vi "Calibration.vi"() -> ()   [LabVIEW 2014]
uses:
  <vilib>/vision/Vision Builder AI/API.llb/IVB Interface - VBAI Version.ctl
panel:
  out "error out":errorcluster
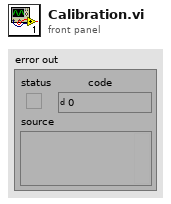
[diagram p1: front panel]
types:
  T1 = typedef "IVB Interface - VBAI Version.ctl" = u16
  T2 = enum32{"invalid app kind", "Development System", "Run Time System", "Student Edition", "Embedded LabVIEW", "Evaluation", "Custom"}
  T3 = typedef "VBAIInterface.ctl" = refnum<k21>
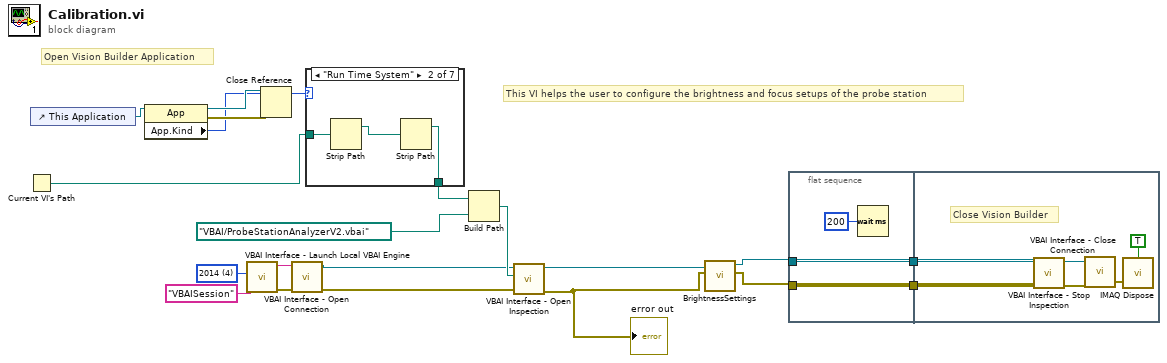
[diagram p0: block diagram]
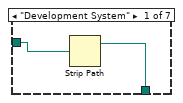
[diagram p2: hidden frame]
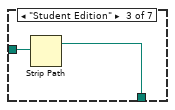
[diagram p3: hidden frame]
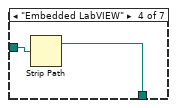
[diagram p4: hidden frame]
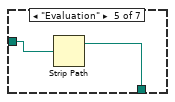
[diagram p5: hidden frame]
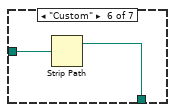
[diagram p6: hidden frame]
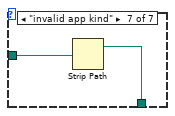
[diagram p7: hidden frame]
diagram:
  w20 = T1 4 items=["2010", "2011", "2012", "2013", "2014"] ("Engine Version")
  # "This VI helps the user to configure the brightness and focus setups of the probe station"
  # "Open Vision Builder Application"
  n1 = Current VI's Path() -> (path=w8:path)
  n2 = control-ref of="This Application"() -> (w10:refnum<vi>)
  n3 = property class="App"(reference=w10) -> (reference out=w12:refnum<vi>, error out=w11:errorcluster, "App.Kind"=w9:T2)  [unwired: 1 in]
  n4 = call <vilib>:"VBAI Interface - Launch Local VBAI Engine.vi"("Engine Version"=w20, "Local VBAI Engine Name"="VBAISession") -> ("error out"=w19:errorcluster, "Session Name Out"=w18:string)  [unwired: 8 in]
  n5 = Close Reference(reference=w12, error in (no error)=w11) -> ()  [unwired: 1 out]
  n6 = call <vilib>:"VBAI Interface - Open Connection.vi"("error in"=w19, "Session In"=w18) -> ("error out"=w13:errorcluster, "Session Out"=w14:T3)  [unwired: 8 in]
  n7 = case shown="\"Run Time System\"" w9 {
    tunnel: w8 -> [w22 w25 w27 w29 w31 w33 w34]
    tunnel: [w21 w23 w26 w28 w30 w32 w35] -> w7
    frame "Development System" {
      n8 = Strip Path(path=w22) -> (stripped path=w21:path)  [unwired: 1 out]
    }
    frame "Run Time System" {
      n9 = Strip Path(path=w25) -> (stripped path=w24:path)  [unwired: 1 out]
      n10 = Strip Path(path=w24) -> (stripped path=w23:path)  [unwired: 1 out]
    }
    frame "Student Edition" {
      n11 = Strip Path(path=w27) -> (stripped path=w26:path)  [unwired: 1 out]
    }
    frame "Embedded LabVIEW" {
      n12 = Strip Path(path=w29) -> (stripped path=w28:path)  [unwired: 1 out]
    }
    frame "Evaluation" {
      n13 = Strip Path(path=w31) -> (stripped path=w30:path)  [unwired: 1 out]
    }
    frame "Custom" {
      n14 = Strip Path(path=w33) -> (stripped path=w32:path)  [unwired: 1 out]
    }
    frame "invalid app kind" {
      n15 = Strip Path(path=w34) -> (stripped path=w35:path)  [unwired: 1 out]
    }
  }
  n16 = Build Path(base path=w7, name or relative path=path "VBAI/ProbeStationAnalyzerV2.vbai") -> (appended path=w15:path)
  n17 = call <vilib>:"VBAI Interface - Open Inspection.vi"("error in"=w13, "Path"=w15, "Session In"=w14) -> ("error out"=w1:errorcluster, "Session Out"=w4:T3)  [unwired: 7 in]
  "error out" <- w1
  n18 = call "BrightnessSettings.vi"("error in (no error)"=w1, "Refnum in"=w4) -> ("error out"=w3:errorcluster, "Refnum out"=w2:T3)  [unwired: 8 in]
  n19 = flat-sequence {
    tunnel: w3 -> [w37]
    tunnel: w2 -> [w38]
    tunnel: [w38] -> w6
    tunnel: [w37] -> w5
    tunnel: w6 -> [w40]
    tunnel: w5 -> [w39]
    frame #0 {
      n20 = Wait (ms)(milliseconds to wait=u32 200) -> ()  [unwired: 1 out]
    }
    frame #1 {
      # "Close Vision Builder"
      n21 = call <vilib>:"VBAI Interface - Stop Inspection.vi"("error in"=w39, "Session In"=w40) -> ("error out"=w41:errorcluster, "Session Out"=w42:T3)  [unwired: 8 in]
      n22 = call <vilib>:"VBAI Interface - Close Connection.vi"("error in"=w41, "Session In"=w42) -> ("error out"=w43:errorcluster)  [unwired: 9 in]
      n23 = call "IMAQ Dispose"("All Images? (No)"=TRUE, "error in (no error)"=w43) -> ()  [unwired: 4 in, 1 out]
    }
  }
